vi "InversePark (FXP).vi"(2 "Theta":fxp<+/-,32,1>, 3 "d":fxp<+/-,32,4>, 4 "q":fxp<+/-,32,12>) -> (0 "beta":fxp<+/-,32,12> format="%.24g", 1 "alpha":fxp<+/-,32,12> format="%.24g")   [LabVIEW 2025]
uses:
  <vilib>/rvi/FXPMathLib/FxpSinAndCos/subVIs/nifxpmath_SinAndCos_SimConfig.ctl
  <vilib>/rvi/FXPMathLib/FxpSinAndCos/simVIs/DllFxpSinAndCosTemp_sub.vi
  <vilib>/rvi/FXPMathLib/FxpSinAndCos/XNode/nifxpmath_SinAndCos.xnode
  <vilib>/rvi/FXPMathLib/FxpAdd/XNode/nifxpmath_Add.xnode
  <vilib>/rvi/FXPMathLib/sim/FxpSim.dll
  <vilib>/rvi/FXPMathLib/FxpMul/XNode/nifxpmath_Multiplier.xnode
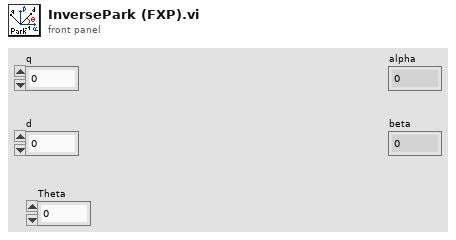
[diagram p1: front panel]
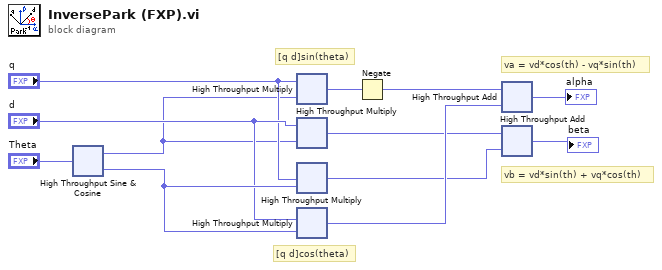
[diagram p0: block diagram]
diagram:
  # "vb = vd*sin(th) + vq*cos(th)"
  # "va = vd*cos(th) - vq*sin(th)"
  # "[q d]cos(theta)"
  # "[q d]sin(theta)"
  n1 = xnode "High Throughput Sine & Cosine"("x (pi)"="Theta") -> ("sin(x)"=w3:fxp<+/-,16,2>, "cos(x)"=w8:fxp<+/-,16,2>)
  n2 = xnode "High Throughput Multiply"("x"="q", "y"=w3) -> ("x*y"=w12:fxp<+/-,32,12>)
  n3 = xnode "High Throughput Multiply"("x"="d", "y"=w3) -> ("x*y"=w4:fxp<+/-,32,12>)
  n4 = xnode "High Throughput Multiply"("x"="q", "y"=w8) -> ("x*y"=w6:fxp<+/-,32,12>)
  n5 = xnode "High Throughput Multiply"("x"="d", "y"=w8) -> ("x*y"=w9:fxp<+/-,32,12>)
  n6 = Negate(x=w12) -> (-x=w1:fxp<+/-,33,13>)
  n7 = xnode "High Throughput Add"("x"=w1, "y"=w9) -> ("x+y"=→"alpha":fxp<+/-,32,12>)
  n8 = xnode "High Throughput Add"("x"=w4, "y"=w6) -> ("x+y"=→"beta":fxp<+/-,32,12>)
